vi "Set Column Widths.vi"(7 "Column Widths":i32[](array[numeric]), 8 "error in (no error)":errorcluster, 10 "Sheet Reference":refnum<k24>) -> (0 "error out":errorcluster, 2 "Sheet Reference out":refnum<k24>)   [LabVIEW 2014]
uses:
  C:/Users/LENOVO/Desktop/CodeSpace GUI/LVExcel/Resources/NPOI.dll
  Resources/NPOI.dll
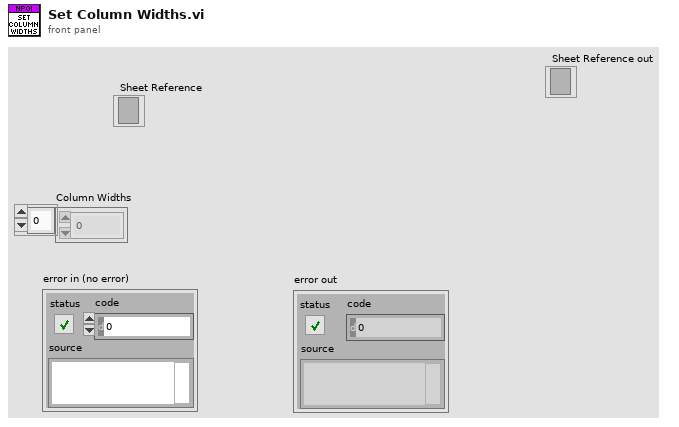
[diagram p1: front panel]
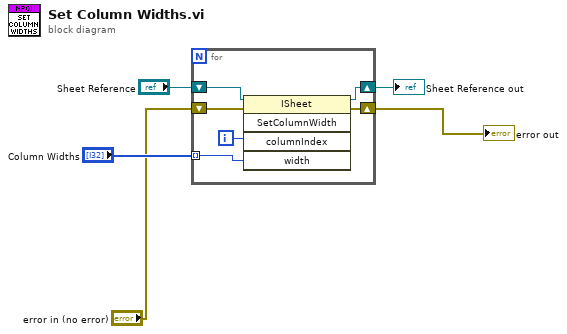
[diagram p0: block diagram]
diagram:
  n1 = for {
    shift-right: [w9] -> w3
    shift-left: "Sheet Reference" -> [w11]
    shift-right: [w8] -> w1
    shift-left: "error in (no error)" -> [w10]
    tunnel: "Column Widths" -> [w6] mode=indexing
    i -> [w7]
    n2 = invoke class="ISheet" method="SetColumnWidth"(reference=w11, error in=w10, "columnIndex"=w7, "width"=w6) -> (reference out=w9:refnum<k24>, error out=w8:errorcluster)  [unwired: 1 in, 3 out]
  }
  "Sheet Reference out" <- w3
  "error out" <- w1
